vi "12bit_2sComplement_single.vi"(1 "Binary in":i16=2057 format="%012b", 2 "Bit Depth":u16=16) -> (0 "Decimal":i16)   [LabVIEW 2012]
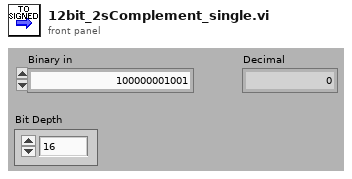
[diagram p1: front panel]
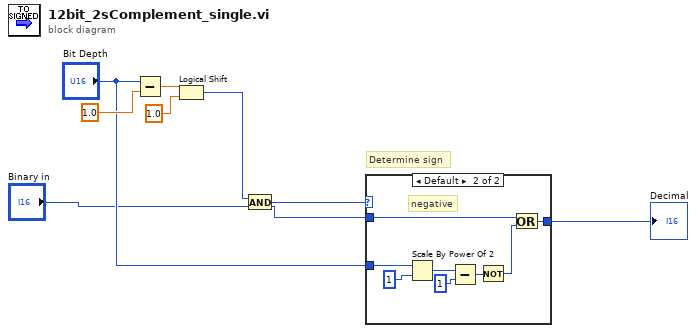
[diagram p0: block diagram]
diagram:
  # "Determine sign"
  n1 = Subtract(x="Bit Depth", y=1.0) -> (x-y=w6:dbl)
  n2 = Logical Shift(y=w6, x=1.0) -> (x << y=w4:u32)
  n3 = And(x=w4, y="Binary in") -> (x .and. y?=w8:u32)
  n4 = case shown="Default" w8 {
    tunnel: [w9 w16] -> w1
    tunnel: "Binary in" -> [w9 w17]
    tunnel: "Bit Depth" -> [_ w14]
    frame 0 {
      # "positive"
    }
    frame Default {
      # "negative"
      n5 = Scale By Power Of 2(n=w14, x=u16 1) -> (x*2^n=w13:u16)
      n6 = Subtract(x=w13, y=u16 1) -> (x-y=w11:u16)
      n7 = Not(x=w11) -> (.not. x?=w10:u16)
      n8 = Or(x=w17, y=w10) -> (x .or. y?=w16:u16)
    }
  }
  "Decimal" <- w1
